vi "Recompose VI.vi"(5 "FPH_/BDH_ (88=X)":u8=88, 6 "Other resources (default)":T1, 7 "Open VI? (F)":bool, 8 "Error in":errorcluster caption="Error in (no error)", 9 "Block Diagram XML":string, 10 "Front Panel XML":string, 11 "Target path (temporary file)":path=path "") -> (0 "Error out":errorcluster, 2 "VI Refnum (if opened)":refnum<vi>, 3 "Target path out":path)   [LabVIEW 2023, in "Resource Manipulation.lvlib"]
uses:
  Resource Manipulation.lvlib
  Resource Array.ctl
  Resource.ctl
  Blank VI.vi
  Find First Matching Resource (String).vi
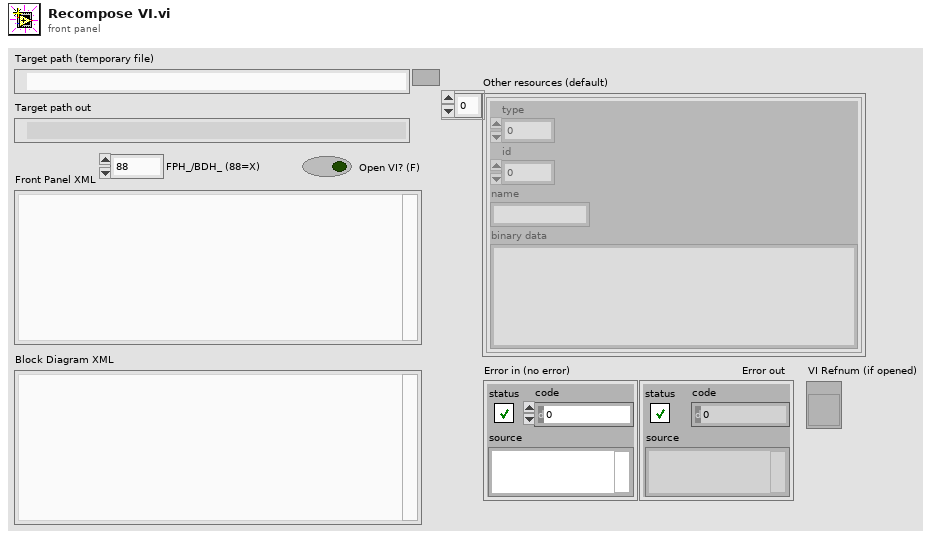
[diagram p1: front panel]
types:
  T1 = typedef "Resource Manipulation.lvlib/Resource Array.ctl" = T2[]
  T2 = typedef "Resource Manipulation.lvlib/Resource.ctl" = cluster{"type":u32, "id":i32, "name":string, "binary data":string}
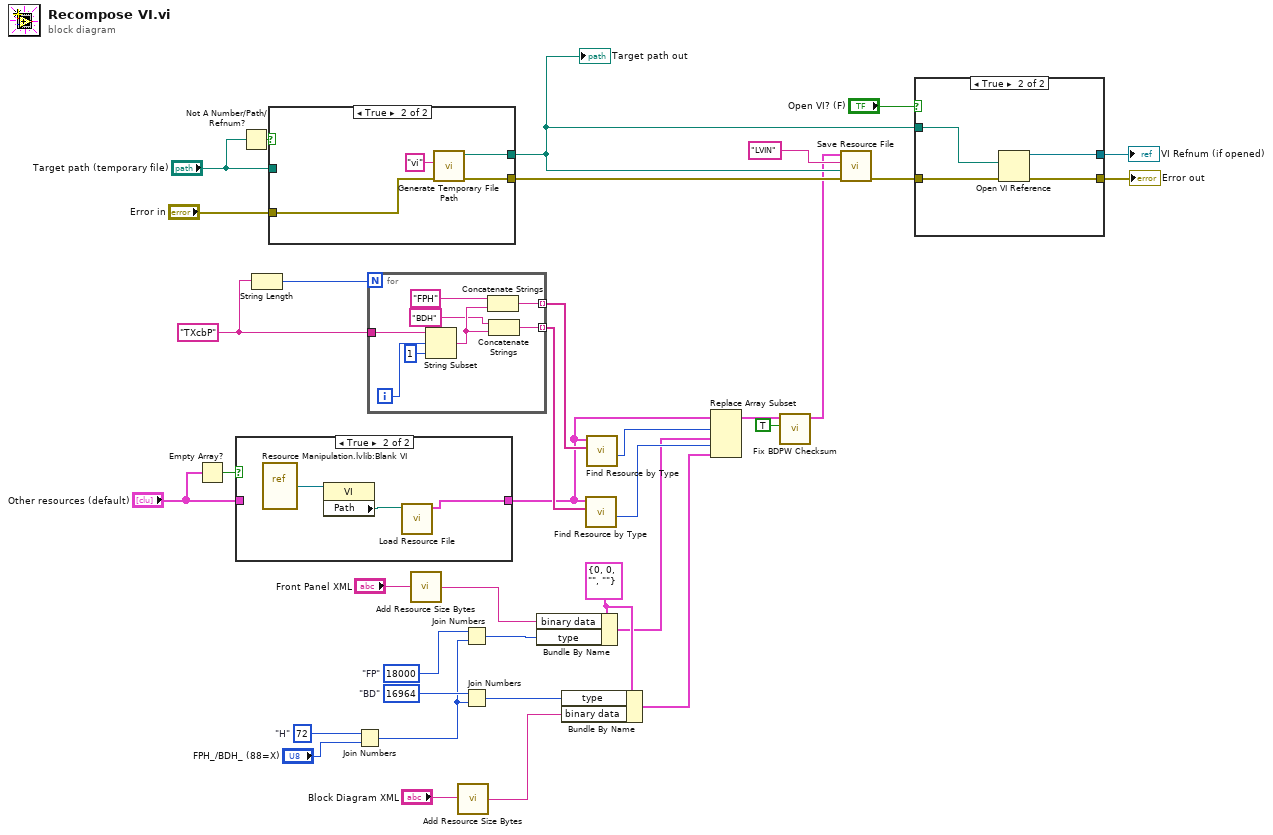
[diagram p0: block diagram]
diagram:
  w14 = u16 18000  # "FP"
  w15 = u16 16964  # "BD"
  w13 = u8 72  # "H"
  w18 = T2 {"type"=0, "id"=0, "name"="", "binary data"=""} ("resource info")
  w32 = "TXcbP"
  n1 = Empty Array?(array="Other resources (default)") -> (empty?=w4:bool)
  n2 = case shown="True" w4 {
    tunnel: "Other resources (default)" -> [w37 _]
    tunnel: [w37 w38] -> w6
    frame False {
    }
    frame True {
      n3 = vi-ref "Resource Manipulation.lvlib:Blank VI.vi"() -> (w40:refnum<vi>)
      n4 = property class="VI"(reference=w40) -> ("Path"=w39:path)  [unwired: 1 in, 2 out]
      n5 = call "Load Resource File.vi"("Resource file"=w39) -> ("Resources"=w38:T1)  [unwired: 8 in, 2 out]
    }
  }
  n6 = Not A Number/Path/Refnum?(number/path/refnum="Target path (temporary file)") -> (NaN/Path/Refnum?=w36:bool)
  n7 = String Length(string=w32) -> (length=w33:i32)
  n8 = case shown="True" w36 {
    tunnel: "Target path (temporary file)" -> [w42 _]
    tunnel: "Error in" -> [w41 w45]
    tunnel: [w41 w44] -> w29
    tunnel: [w42 w43] -> w23
    frame False {
    }
    frame True {
      n9 = call <vilib>:"Generate Temporary File Path.vi"("error in (no error)"=w45, "Temporary File Extension (tmp)"="vi") -> ("error out"=w44:errorcluster, "Unique Temporary File Path"=w43:path)  [unwired: 8 in]
    }
  }
  "Target path out" <- w23
  n10 = Join Numbers(hi=w13, lo="FPH_/BDH_ (88=X)") -> ((hi.lo)=w11:u16)
  n11 = for {
    N: w33 -> [_]
    tunnel: w32 -> [w54]
    tunnel: [w48] -> w30 mode=indexing
    tunnel: [w47] -> w31 mode=indexing
    i -> [w53]
    n12 = String Subset(string=w54, offset (0)=w53, length (rest)=1 ("length (rest)")) -> (substring=w51:string)
    n13 = Concatenate Strings("FPH", w51) -> (w48:string)
    n14 = Concatenate Strings("BDH", w51) -> (w47:string)
  }
  n15 = call "Add Resource Size Bytes.vi"("Data In"="Front Panel XML") -> ("Data Out"=w9:string)
  n16 = call "Add Resource Size Bytes.vi"("Data In"="Block Diagram XML") -> ("Data Out"=w7:string)
  n17 = Join Numbers(hi=w14, lo=w11) -> ((hi.lo)=w20:u32)
  n18 = Join Numbers(hi=w15, lo=w11) -> ((hi.lo)=w19:u32)
  n19 = Bundle By Name(cluster=w18, "binary data"=w9, "type"=w20) -> (w17:T2)
  n20 = Bundle By Name(cluster=w18, "type"=w19, "binary data"=w7) -> (w16:T2)
  n21 = call-poly "Find Resource by Type.vi"("Resource Types"=w31, "Resources"=w6) -> ("Index"=w26:i32)  [unwired: 6 in, 3 out]
  n22 = call-poly "Find Resource by Type.vi"("Resource Types"=w30, "Resources"=w6) -> ("Index"=w27:i32)  [unwired: 6 in, 3 out]
  n23 = Replace Array Subset(array=w6, new element #1=w17, index #1=w27, new element #2=w16, index #2=w26) -> (w3:T1)
  n24 = call "Fix BDPW Checksum.vi"("Only fix 3rd hash (F)"=TRUE, "Resources in"=w3) -> ("Resources out"=w2:T1)  [unwired: 9 in]
  n25 = call "Save Resource File.vi"("error in (no error)"=w29, "Path"=w23, "File type"="LVIN", "Resources"=w2) -> ("error out"=w24:errorcluster)  [unwired: 7 in]
  n26 = case shown="True" "Open VI? (F)" {
    tunnel: w24 -> [w55 w59]
    tunnel: w23 -> [_ w58]
    tunnel: [_ w57] -> w22
    tunnel: [w55 w56] -> w21
    frame False {
    }
    frame True {
      n27 = Open VI Reference(vi path=w58, error in (no error)=w59) -> (vi reference=w57:refnum<vi>, error out=w56:errorcluster)  [unwired: 4 in]
    }
  }
  "Error out" <- w21
  "VI Refnum (if opened)" <- w22
